vi "Img_msg_ex.vi"(1 "Msg Type":T2, 3 "Message In":string="dfsdfgsdfgdfg\r Saved in DB") -> (0 "Message":picture)   [LabVIEW 2020]
uses:
  Controls/Msg_Type.ctl
  <vilib>/picture/picture.llb/Draw True-Color Pixmap.vi
panel:
  out "text rect":T1
  out "after substring":string
  out "trimmed string":string
  out "element":string
  out "new picture 2":picture
  out "new picture":picture
  # "29032640/DC1343Bf000031\\rPASS\\sSaved\\sin\\sDB"
  # "Incorrect PKYK RFID Tag"
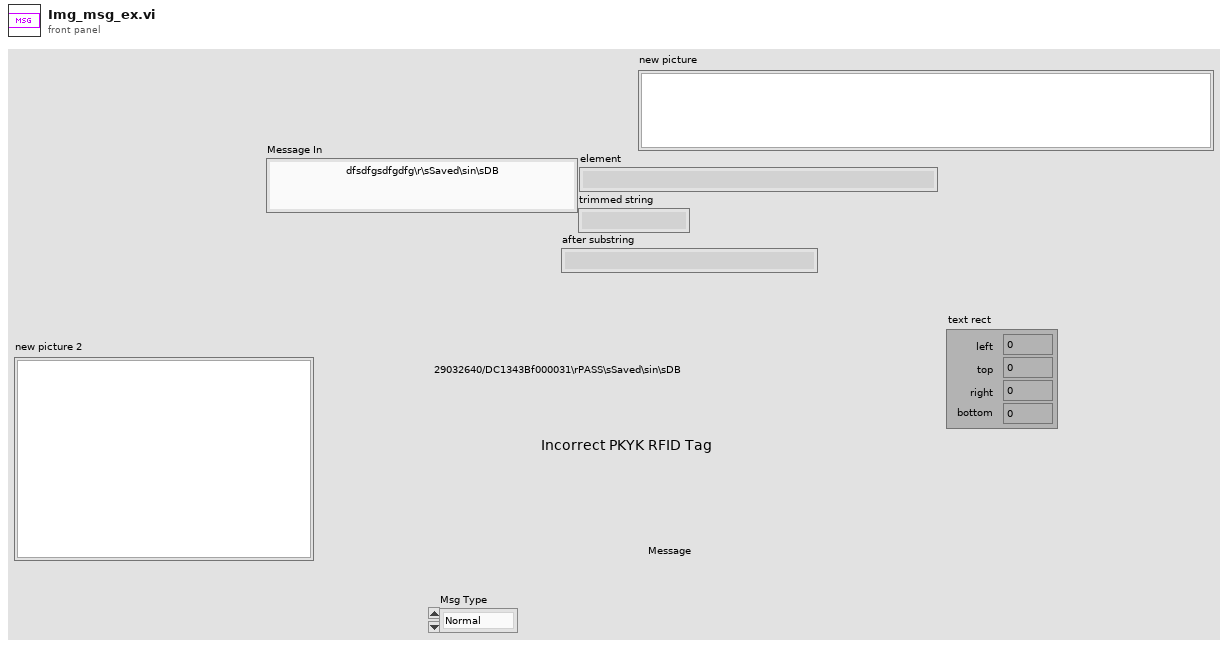
[diagram p1: front panel]
types:
  T1 = cluster{"left":i16, "top":i16, "right":i16, "bottom":i16}
  T2 = typedef "Msg_Type.ctl" = enum16{"Normal", "Pass", "Fail", "Fault", "User", "Bypass", "Fail Save"}
  T3 = cluster{"left":i16, "top":i16, "right":i16, "bottom":dbl}
  T4 = enum16{"None", "Stacked", "Clockwise", "Counterclockwise"}
  T5 = cluster{"Font Name:":string, "Size":i16, "Strikeout?":bool, "Italic?":bool, "Underline?":bool, "Outline?":bool, "Shadow?":bool, "Bold?":bool}
  T6 = enum16{"User-specified Font", "Application Font", "System Font", "Dialog Font"}
  T7 = typedef "imagedata.ctl" = cluster{"image type":i32, "image depth":i32, "image":u8[], "mask":u8[], "colors":u32[], "Rectangle":cluster{"left":i16, "top":i16, "right":i16, "bottom":i16}}
  T8 = cluster{"left":dbl, "top":dbl, "right":dbl, "bottom":dbl}
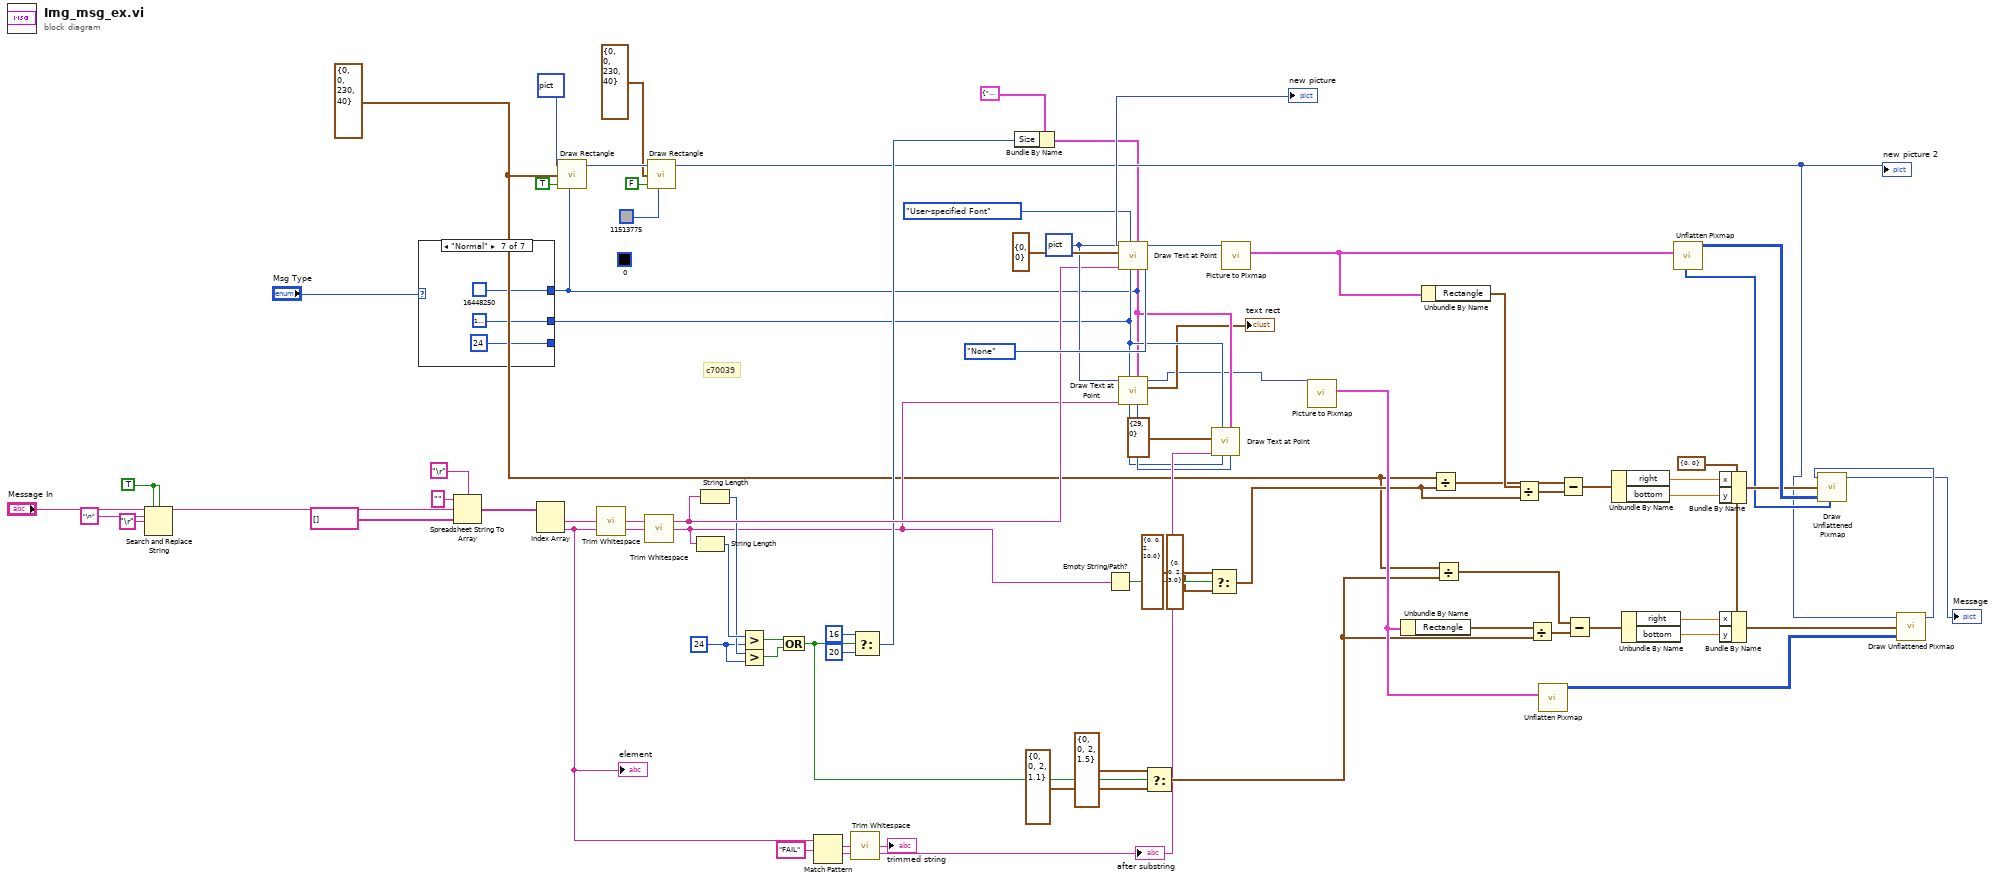
[diagram p0: block diagram]
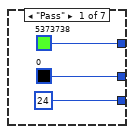
[diagram p2: hidden frame]
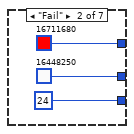
[diagram p3: hidden frame]
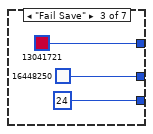
[diagram p4: hidden frame]
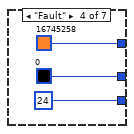
[diagram p5: hidden frame]
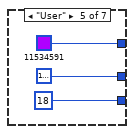
[diagram p6: hidden frame]
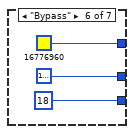
[diagram p7: hidden frame]
diagram:
  w2 = T1 {"left"=0, "top"=0, "right"=230, "bottom"=40} ("output cluster")
  (unwired) u32 0 ("color(black)")
  w23 = TRUE ("replace all? (F)")
  w33 = 24 ("y")
  w51 = cluster{"x":i16, "y":i16} {"x"=0, "y"=0} ("top left point(0, 0)")
  w11 = T6."User-specified Font" ("desired font(Application)")
  w52 = picture data[5B] ("picture")
  # "c70039"
  n1 = Search and Replace String(replace all?=w23, case sensitive?=w23, input string="Message In", search string="\n", replace string="\r" ("replace string (\"\")")) -> (result string=w24:string)  [unwired: 3 in, 3 out]
  n2 = case shown="\"Normal\"" "Msg Type" {
    tunnel: [u32 5373738 ("color(black)") u32 16711680 ("color(black)") u32 13041721 ("color(black)") u32 16745258 ("color(black)") u32 11534591 ("color(black)") u32 16776960 ("color(black)") u32 16448250 ("color(black)")] -> w4
    tunnel: [u32 0 ("color(black)") u32 16448250 ("color(black)") u32 16448250 ("color(black)") u32 0 ("color(black)") u32 16777226 ("color(black)") u32 16777222 ("color(black)") u32 16777222 ("color(black)")] -> w3
    tunnel: [i16 24 ("Size") i16 24 ("Size") i16 24 ("Size") i16 24 ("Size") i16 18 ("Size") i16 18 ("Size") i16 24 ("Size")] -> _
    frame "Pass" {
    }
    frame "Fail" {
    }
    frame "Fail Save" {
    }
    frame "Fault" {
    }
    frame "User" {
    }
    frame "Bypass" {
    }
    frame "Normal" {
    }
  }
  n3 = Spreadsheet String To Array(delimiter (Tab)="\r", format string="", spreadsheet string=w24, array type (2D Dbl)=string[] []) -> (array=w54:string[])
  n4 = Index Array(array=w54) -> (element #1=w53:string, element #2=w14:string)  [unwired: 2 in]
  "element" <- w14
  n5 = call <vilib>:"Draw Rectangle.vi"("picture"=picture data[5B], "rect"=w2, "fill?(F)"=TRUE, "color(black)"=w4) -> ("new picture"=w73:picture)  [unwired: 5 in]
  n6 = call <vilib>:"Trim Whitespace.vi"("string"=w53) -> ("trimmed string"=w36:string)  [unwired: 1 in]
  n7 = call <vilib>:"Trim Whitespace.vi"("string"=w14) -> ("trimmed string"=w5:string)  [unwired: 1 in]
  n8 = call <vilib>:"Draw Rectangle.vi"("picture"=w73, "rect"=T1 {"left"=0, "top"=0, "right"=230, "bottom"=40} ("output cluster"), "fill?(F)"=FALSE, "color(black)"=u32 11513775) -> ("new picture"=w22:picture)  [unwired: 5 in]
  "new picture 2" <- w22
  n9 = String Length(string=w5) -> (length=w35:i32)
  n10 = String Length(string=w36) -> (length=w34:i32)
  n11 = Greater?(x=w35, y=w33) -> (0:w32:bool)
  n12 = Greater?(x=w34, y=w33) -> (0:w31:bool)
  n13 = Compound Arithmetic op=OR(w32, w31) -> (w19:bool)
  n14 = Match Pattern(string=w14, regular expression="FAIL") -> (match substring=w15:string, after substring=w9:string)  [unwired: 1 in, 2 out]
  "after substring" <- w9
  n15 = call <vilib>:"Trim Whitespace.vi"("string"=w15) -> ("trimmed string"=→"trimmed string":string)  [unwired: 1 in]
  n16 = Select(t=i16 16, s=w19, f=i16 20 ("Size")) -> (s? t:f=w28:i16)
  n17 = Bundle By Name(cluster=T5 {"Font Name:"="Segoe UI Semibold", "Size"=18, "Strikeout?"=FALSE, "Italic?"=FALSE, "Underline?"=FALSE, "Outline?"=FALSE, "Shadow?"=FALSE, "Bold?"=FALSE} ("[user-specified font]"), "Size"=w28) -> (w10:T5)
  n18 = Empty String/Path?(string/path=w5) -> (empty?=w40:bool)
  n19 = call <vilib>:"Draw Text at Point.vi"("text orientation"=T4."None", "BG color(transparent)"=w4, "[user-specified font]"=w10, "text color(black)"=w3, "desired font(Application)"=w11, "text"=w36, "origin"=cluster{"x":i16, "y":i16} {"x"=0, "y"=0}, "picture"=w52) -> ("new picture"=w69:picture)  [unwired: 2 in, 1 out]
  "new picture" <- w69
  n20 = call <vilib>:"Draw Text at Point.vi"("BG color(transparent)"=w4, "[user-specified font]"=w10, "text color(black)"=w3, "desired font(Application)"=w11, "text"=w5, "picture"=w52) -> ("text rect"=→"text rect":T1, "new picture"=w6:picture)  [unwired: 4 in]
  n21 = Select(t=T3 {"left"=0, "top"=0, "right"=2, "bottom"=1.5} ("output cluster 2"), s=w19, f=T3 {"left"=0, "top"=0, "right"=2, "bottom"=1.1} ("output cluster 2")) -> (s? t:f=w16:T3)
  n22 = Select(t=T3 {"left"=0, "top"=0, "right"=2, "bottom"=3.0} ("output cluster"), s=w40, f=T3 {"left"=0, "top"=0, "right"=2, "bottom"=10.0} ("output cluster")) -> (s? t:f=w37:T3)
  n23 = call <vilib>:"Draw Text at Point.vi"("BG color(transparent)"=w4, "[user-specified font]"=w10, "text color(black)"=w3, "desired font(Application)"=w11, "text"=w9, "origin"=cluster{"x":i16, "y":i16} {"x"=29, "y"=0}) -> ()  [unwired: 4 in, 2 out]
  n24 = call <vilib>:"Picture to Pixmap.vi"("picture"=w69) -> ("image data"=w60:T7)  [unwired: 9 in, 1 out]
  n25 = call <vilib>:"Picture to Pixmap.vi"("picture"=w6) -> ("image data"=w47:T7)  [unwired: 9 in, 1 out]
  n26 = Unbundle By Name(w47) -> ("Rectangle"=w43:T1)
  n27 = Unbundle By Name(w60) -> ("Rectangle"=w67:T1)
  n28 = Divide(x=w2, y=w37) -> (x/y=w66:T8)
  n29 = Divide(x=w2, y=w16) -> (x/y=w41:T8)
  n30 = Divide(x=w67, y=w37) -> (x/y=w65:T8)
  n31 = Divide(x=w43, y=w16) -> (x/y=w42:T8)
  n32 = call <vilib>:"Unflatten Pixmap.vi"("image data"=w47) -> ("24-bit pixmap"=w46:u32[][])  [unwired: 4 in, 6 out]
  n33 = Subtract(x=w66, y=w65) -> (x-y=w45:T8)
  n34 = Subtract(x=w41, y=w42) -> (x-y=w44:T8)
  n35 = Unbundle By Name(w45) -> ("right"=w63:dbl, "bottom"=w62:dbl)
  n36 = Unbundle By Name(w44) -> ("right"=w50:dbl, "bottom"=w49:dbl)
  n37 = call <vilib>:"Unflatten Pixmap.vi"("image data"=w60) -> ("24-bit pixmap"=w68:u32[][], "mask"=w61:u8[])  [unwired: 4 in, 5 out]
  n38 = Bundle By Name(cluster=w51, "x"=w63, "y"=w62) -> (w64:cluster{"x":i16, "y":i16})
  n39 = Bundle By Name(cluster=w51, "x"=w50, "y"=w49) -> (w48:cluster{"x":i16, "y":i16})
  n40 = call-poly <vilib>:"Draw Unflattened Pixmap.vi"("picture"=w22, "top left point(0, 0)"=w48, "data (RGB format)"=w46) -> ("new picture"=w21:picture)  [unwired: 6 in]
  n41 = call-poly <vilib>:"Draw Unflattened Pixmap.vi"("picture"=w21, "top left point(0, 0)"=w64, "data (RGB format)"=w68, "mask"=w61) -> ("new picture"=→"Message":picture)  [unwired: 5 in]
